vi "Modbus_Decode_Multiple_registers.vi"(10 "Temp. unit:":u16, 11 "register values":u16[](array[numeric])) -> (1 "Numeric 3":dbl, 2 "Numeric 4":dbl, 3 "Numeric 5":dbl, 4 "Numeric 2":dbl, 5 "register":u16, 6 "Numeric":dbl)   [LabVIEW 2020]
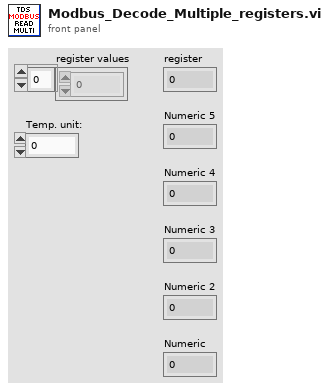
[diagram p1: front panel]
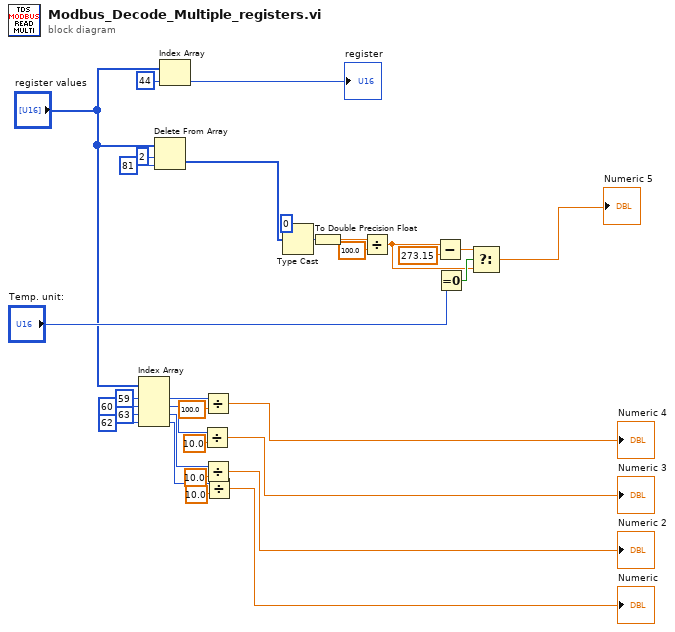
[diagram p0: block diagram]
diagram:
  n1 = Index Array(array="register values", index #1=59 ("index"), index #2=60 ("index"), index #3=63 ("index"), index #4=62 ("index")) -> (element #1=w21:u16, element #2=w25:u16, element #3=w26:u16, element #4=w27:u16)
  n2 = Delete From Array(array="register values", length=2, index=81) -> (deleted portion=w5:u16[])  [unwired: 1 out]
  n3 = Index Array(array="register values", index=44) -> (element=→"register":u16)
  n4 = Divide(x=w25, y=10.0) -> (x/y=→"Numeric 3":dbl)
  n5 = Divide(x=w21, y=100.0) -> (x/y=→"Numeric 4":dbl)
  n6 = Divide(x=w26, y=10.0) -> (x/y=→"Numeric 2":dbl)
  n7 = Divide(x=w27, y=10.0) -> (x/y=→"Numeric":dbl)
  n8 = Type Cast(type=0, x=w5) -> (*(type *) &x=w6:i32)
  n9 = To Double Precision Float(number=w6) -> (double precision float=w12:dbl)
  n10 = Divide(x=w12, y=100.0) -> (x/y=w8:dbl)
  n11 = Subtract(x=w8, y=273.15) -> (x-y=w10:dbl)
  n12 = Equal To 0?(x="Temp. unit:") -> (x = 0?=w32:bool)
  n13 = Select(t=w10, s=w32, f=w8) -> (s? t:f=→"Numeric 5":dbl)
